vi "Transform And Project.vi"(11 "Scene in":refnum<class "Scene.lvclass">) -> (3 "Scene out":refnum<class "Scene.lvclass">)   [LabVIEW 2020, in "Scene.lvclass"]
uses:
  Scene.lvclass
  Scene.lvclass/Scene.ctl
  196e4586-e654-41ec-a3a4-43fea5068e8e.vi
  Graphics/Libraries/3D/Vector 3D.ctl
  Graphics/Libraries/3D/3D.lvlib
  a59a4b44-279f-4314-be75-e28f6a03f0ec.vi
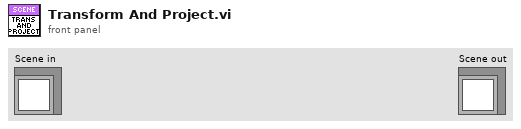
[diagram p1: front panel]
types:
  T1 = typedef "3D.lvlib/Vector 3D.ctl" = cluster{"x":sgl, "y":sgl, "z":sgl}
  T2 = typedef "Raster.lvlib/Rectangle Dimensions.ctl" = cluster{"Width":u32, "Height":u32}
  T3 = typedef "3D.lvlib/Object.ctl" = cluster{"Triangles":T4[], "Transform":T9, "Name":string, "Alpha Blending Enabled":bool, "Alpha":dbl, "Turntable Enabled":bool, "Material":T7}
  T4 = typedef "3D.lvlib/Triangle.ctl" = cluster{"Vertex 1":T5, "Vertex 2":T5, "Vertex 3":T5, "Alpha":dbl, "Alpha Blending Enabled":bool, "Colour":u32, "Material":T7}
  T5 = typedef "3D.lvlib/Vertex.ctl" = cluster{"Position":T1, "UV":T6, "Colour":u32}
  T6 = typedef "Raster.lvlib/UV.ctl" = cluster{"u":sgl, "v":sgl}
  T7 = typedef "3D.lvlib/Material.ctl" = cluster{"Diffuse Colour":u32, "Texture":T8}
  T8 = typedef "Raster.lvlib/Texture.ctl" = cluster{"Pixels":refnum<data-value>, "Size":T2}
  T9 = typedef "3D.lvlib/Transform.ctl" = cluster{"Position":T1, "Rotation":T1, "Scale":T1}
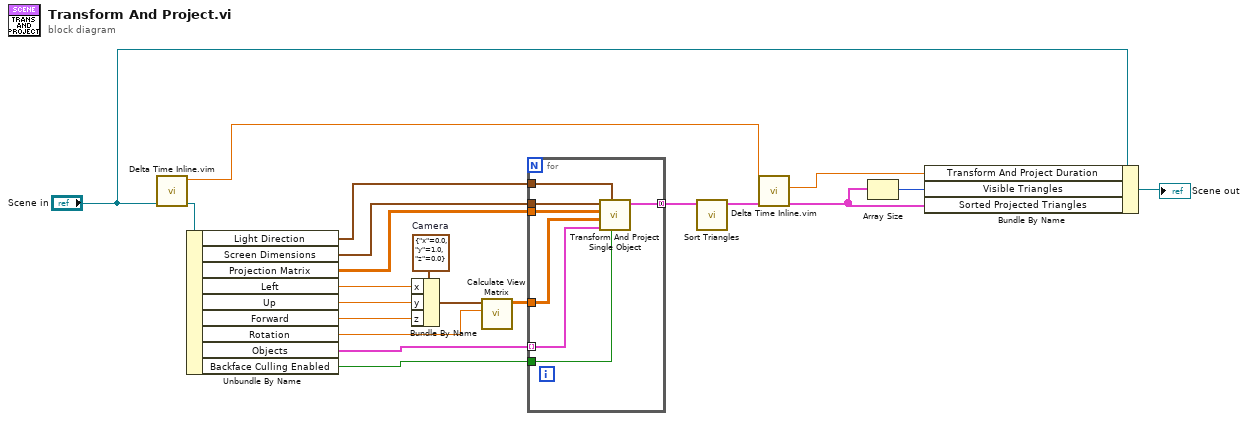
[diagram p0: block diagram]
diagram:
  w20 = T1 {"x"=0.0, "y"=1.0, "z"=0.0}  # Camera
  n1 = call "Delta Time Inline.vim"("value in"="Scene in") -> ("value out"=w21:refnum<class "Scene.lvclass">, "Relative Seconds out [s]"=w13:dbl)  [unwired: 8 in, 1 out]
  n2 = Unbundle By Name(w21) -> ("Light Direction"=w2:T1, "Screen Dimensions"=w4:T2, "Projection Matrix"=w3:sgl[][], "Left"=w15:sgl, "Up"=w16:sgl, "Forward"=w19:sgl, "Rotation"=w17:sgl, "Objects"=w5:T3[], "Backface Culling Enabled"=w1:bool)
  n3 = Bundle By Name(cluster=w20, "x"=w15, "y"=w16, "z"=w19) -> (w14:T1)
  n4 = call "Calculate View Matrix.vi"("Camera Rotation"=w17, "Camera Position"=w14) -> ("View Matrix"=w18:sgl[][])  [unwired: 9 in]
  n5 = for {
    tunnel: w18 -> [w25]
    tunnel: [w28] -> w7 mode=concatenating
    tunnel: w5 -> [w24] mode=indexing
    tunnel: w4 -> [w27]
    tunnel: w3 -> [w26]
    tunnel: w2 -> [w23]
    tunnel: w1 -> [w22]
    n6 = call "Transform And Project Single Object.vi"("Backface Culling Enabled"=w22, "Light Direction"=w23, "Object"=w24, "View Matrix"=w25, "Projection Matrix"=w26, "Screen Dimensions"=w27) -> ("Triangles"=w28:T4[])  [unwired: 5 in]
  }
  n7 = call "Sort Triangles.vi"("Triangles"=w7) -> ("Triangles Sorted"=w6:T4[])  [unwired: 10 in]
  n8 = call "Delta Time Inline.vim"("value in"=w6, "Relative Seconds in [s]"=w13) -> ("value out"=w10:T4[], "Delta Time [s]"=w9:dbl)  [unwired: 7 in, 1 out]
  n9 = Array Size(array=w10) -> (size(s)=w8:i32)
  n10 = Bundle By Name(cluster="Scene in", "Transform And Project Duration"=w9, "Visible Triangles"=w8, "Sorted Projected Triangles"=w10) -> (→"Scene out":refnum<class "Scene.lvclass">)
